vi "Graph Cluster.vi"() -> ()   [LabVIEW 2010]
panel:
  in  "stop":bool
  out "Waveform Graph 2":cluster{i32, i32, dbl[]}(graph)
  out "Waveform Graph":dbl[](graph)
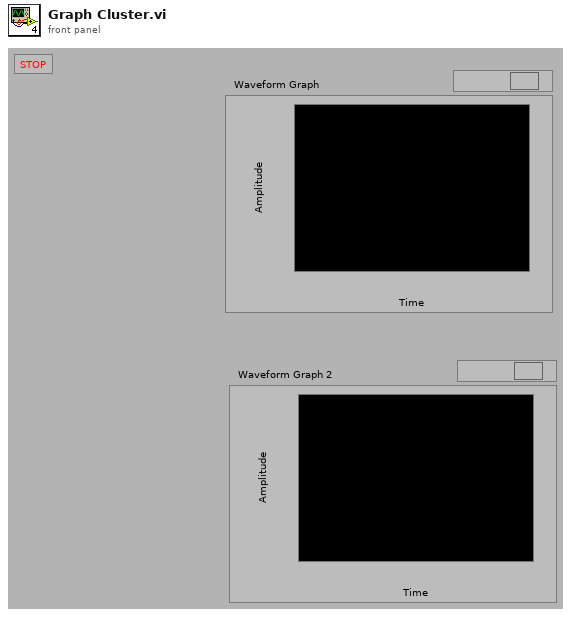
[diagram p1: front panel]
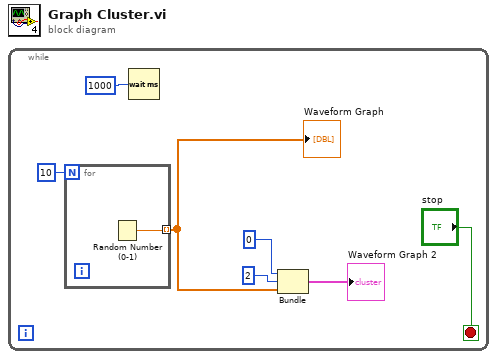
[diagram p0: block diagram]
diagram:
  n1 = while {
    stop <- "stop" stop-if-true
    n2 = for {
      N: 10 -> [_]
      tunnel: [w8] -> w5 mode=indexing
      n3 = Random Number (0-1)() -> (number: 0 to 1=w8:dbl)
    }
    "Waveform Graph" <- w5
    n4 = Wait (ms)(milliseconds to wait=1000) -> ()  [unwired: 1 out]
    n5 = Bundle(0, 2, w5) -> (→"Waveform Graph 2":cluster{i32, i32, dbl[]})  [unwired: 1 in]
  }
